vi "agilent_34970A_votlage.vi"(0 "error in (no error)":errorcluster, 1 "Readings":u16=25, 2 "Channels":string="107", 3 "Agilent Port In":refnum<visa-resource-name>="COM35") -> (6 "error out":errorcluster, 7 "Voltage Standard Deviations":dbl[](array[numeric]) format="%_6f", 8 "Voltage Averages":dbl[](array[numeric]) format="%_6f", 9 "Agilent Port Out":refnum<visa-resource-name>="COM35")   [LabVIEW 2010]
uses:
  <vilib>/Analysis/NI_AALBase.lvlib
panel:
  out "Waveform Graph":dbl[][](graph)
  out "Raw Voltages":dbl[][](array[numeric]) format="%_6f"
  out "Voltages":string
  # "This graph isn't actually required for anything. It could easily be dispensed with."
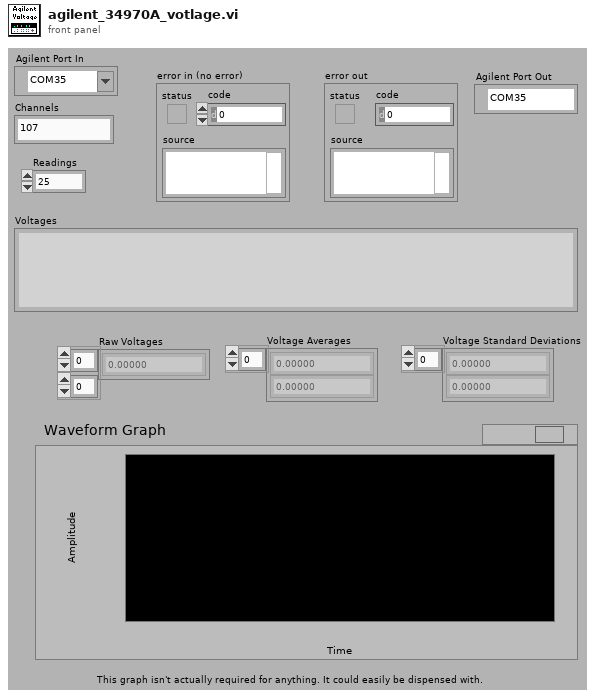
[diagram p1: front panel]
types:
  T1 = enum16{"Enable Register", "Event Register", "Operation Complete Bit"}
  T2 = enum16{"Manual", "Minimum", "Maximum", "Infinity"}
  T3 = enum16{"Bus", "Immediate", "External", "Alarm 1", "Alarm 2", "Alarm 3", "Alarm 4", "Timer"}
  T4 = cluster{"Include Alarm Data? (F:No)":bool, "Include Channel #? (F:No)":bool, "Include Time? (F:No)":bool, "Include Units? (F:No)":bool}
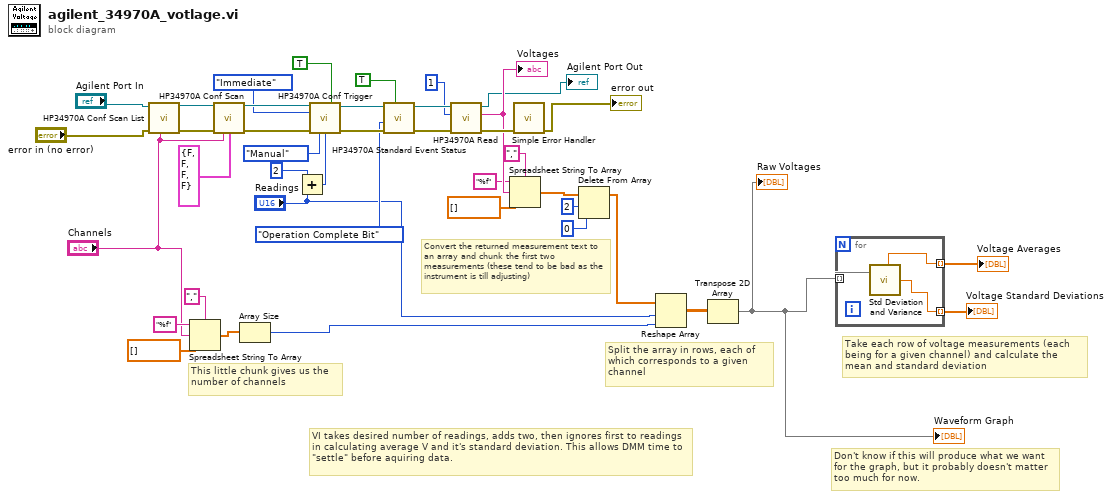
[diagram p0: block diagram]
diagram:
  # "Convert the returned measurement text to an array and chunk the first two measurements (these tend to be bad as the instrument is till adjusting)"
  # "Don't know if this will produce what we want for the graph, but it probably doesn't matter too much for now."
  # "Take each row of voltage measurements (each being for a given channel) and calculate the mean and standard deviation"
  # "Split the array in rows, each of which corresponds to a given channel"
  # "This little chunk gives us the number of channels"
  # "VI takes desired number of readings, adds two, then ignores first to readings in calculating average V and it's standard deviation. This allows DMM time to \"settle\" before aquiring data."
  n1 = call "HP34970A Conf Scan List.vi"("Scan List (empty)"="Channels", "error in (no error)"="error in (no error)", "VISA resource name"="Agilent Port In") -> ("error out"=w37:errorcluster, "VISA resource name out"=w38:refnum<visa-resource-name>)  [unwired: 6 in, 1 out]
  n2 = Spreadsheet String To Array(delimiter (Tab)=",", format string="%f", spreadsheet string="Channels", array type (2D Dbl)=dbl[] []) -> (array=w6:dbl[])
  n3 = call "HP34970A Conf Scan.vi"("VISA resource name"=w38, "error in (no error)"=w37, "Channel List (empty)"="Channels", "Scan Fields"=T4 {"Include Alarm Data? (F:No)"=FALSE, "Include Channel #? (F:No)"=FALSE, "Include Time? (F:No)"=FALSE, "Include Units? (F:No)"=FALSE}) -> ("VISA resource name out"=w35:refnum<visa-resource-name>, "error out"=w34:errorcluster)  [unwired: 9 in, 1 out]
  n4 = Array Size(array=w6) -> (size(s)=w5:i32)
  n5 = Add(x=u16 2, y="Readings") -> (x+y=w19:u16)
  n6 = call "HP34970A Conf Trigger.vi"("VISA resource name"=w35, "Wait for Trigger? (F:No)"=TRUE, "Source (1:Immediate)"=T3."Immediate", "error in (no error)"=w34, "Max Trigger Count (3:Inf)"=T2."Manual", "# Triggers (1)"=w19) -> ("VISA resource name out"=w30:refnum<visa-resource-name>, "error out"=w29:errorcluster)  [unwired: 7 in, 1 out]
  n7 = call "HP34970A Standard Event Status.vi"("Set/Check? (F:Set)"=TRUE, "error in (no error)"=w29, "Check Parameter (0:Enable Reg)"=T1."Operation Complete Bit", "VISA resource name"=w30) -> ("error out"=w40:errorcluster, "VISA resource name out"=w39:refnum<visa-resource-name>)  [unwired: 5 in, 1 out]
  n8 = call "HP34970A Read.vi"("error in (no error)"=w40, "# Channels (1)"=1, "VISA resource name"=w39) -> ("error out"=w41:errorcluster, "Readings"=w24:string, "VISA resource name out"=→"Agilent Port Out":refnum<visa-resource-name>)  [unwired: 5 in, 1 out]
  "Voltages" <- w24
  n9 = Spreadsheet String To Array(delimiter (Tab)=",", format string="%f", spreadsheet string=w24, array type (2D Dbl)=dbl[] []) -> (array=w18:dbl[])
  n10 = call <vilib>:"Simple Error Handler.vi"("error in (no error)"=w41) -> ("error out"=→"error out":errorcluster)  [unwired: 4 in, 4 out]
  n11 = Delete From Array(array=w18, length=2, index=0) -> (array with subset deleted=w7:dbl[])  [unwired: 1 out]
  n12 = Reshape Array(w7, "Readings", w5) -> (w8:dbl[][])
  n13 = Transpose 2D Array(2D array=w8) -> (transposed array=w3:dbl[][])
  "Raw Voltages" <- w3
  "Waveform Graph" <- w3
  n14 = for {
    tunnel: w3 -> [w44] mode=indexing
    tunnel: [w43] -> w2 mode=indexing
    tunnel: [w42] -> w1 mode=indexing
    n15 = call <vilib>:"Std Deviation and Variance.vi"("X"=w44) -> ("mean"=w43:dbl, "standard deviation"=w42:dbl)  [unwired: 1 in, 1 out]
  }
  "Voltage Averages" <- w2
  "Voltage Standard Deviations" <- w1
